vi "keithley_237_read_current_86.vi"(2 "error in":T1, 3 "GPIB":string) -> (0 "error out":T1, 1 "Current":dbl)   [LabVIEW 2009]
panel:
  out "status":bool[](array[boolean])=[TRUE]
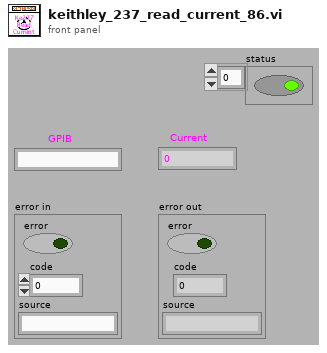
[diagram p1: front panel]
types:
  T1 = cluster{"error":bool, "code":i32, "source":string}
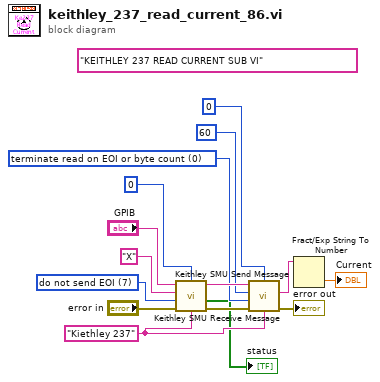
[diagram p0: block diagram]
diagram:
  (unwired) "KEITHLEY 237 READ CURRENT SUB VI"
  w8 = 0 items=["terminate read on EOI or byte count", "terminate read on EOI, byte count, or CR", "terminate read on EOI, byte count, or LF"] ("read mode (EOI:0)")
  w9 = "Kiethley 237" ("source")
  w11 = 7 items=["send EOI with last character of string", "append CR to string and send EOI with CR", "append LF to string and send EOI with LF", "append CR LF to string and send EOI with LF", "append CR to string but do not send EOI", "append LF to string but do not send EOI", "append CR LF to string but do not send EOI", "do not send EOI"] ("write mode (send EOI:0)")
  n1 = call <instrlib>:"Keithley SMU Send Message.vi"("timeout ms"=u32 0, "address string"="GPIB", "write buffer"="X", "source"=w9, "write mode (send EOI:0)"=w11, "error in"="error in") -> ("address out"=w10:string, "status"=→"status":bool[], "error out"=w14:T1)  [unwired: 1 out]
  n2 = call <instrlib>:"Keithley SMU Receive Message.vi"("timeout ms"=u32 0, "address string"=w10, "byte count"=60, "source"=w9, "read mode (EOI:0)"=w8, "error in"=w14) -> ("read buffer"=w4:string, "error out"=→"error out":T1)  [unwired: 2 out]
  n3 = Fract/Exp String To Number(string=w4) -> (number=→"Current":dbl)  [unwired: 3 in, 1 out]
